vi "Close.vi"(8 "error in (no error)":errorcluster, 11 "Pump Calibration Config in":T1={"Settings"={"Cycle Period"=500.0, "Ismatech"={"VISA resource name"="", "Simulated?"=TRUE, "Pump Number"=1.0, "Reverse?"=FALSE}, "Masterflex"={"VISA resource name"="", "Simulated?"=TRUE, "Pump Number"=1.0, "Reverse?"=FALSE}, "Bronkhorst M13 Settings"={"VISA resource name"="", "Simulated?"=TRUE, "Smoothing Steps"=1}, "PID 2 Parameters"={"Input Device"=enum."Default", "Output Device"=enum."Default"}, "Tacmina Settings"={"Analog DAQ Task"="", "Digital DAQ Task"=""}, "KNF SIMDOS Settings"={"VISA resource name"="", "Simulated?"=TRUE}, "VICI M50 Settings"={"VISA resource name"="", "Pump ID"="", "Pump Head Vol"=0.0, "Reverse?"=FALSE, "Simulated?"=TRUE}, "FLOM Settings"={"VISA resource name"="", "Simulated?"=TRUE, "Pump Number"=0.0}, "Calibration Limits"={"Minimum (ml/min)"=0.0, "Maximum (ml/min)"=0.0, "Steps"=0.0}, "SSI PR Settings"={"VISA resource name"="", "Simulated?"=FALSE}, "Ismatech 4308 Settings"={"VISA resource name"="", "Pump Number"=1, "Channel Number"=0, "Simulated?"=TRUE, "Reverse?"=FALSE}, "Bronkhorst M14 Settings"={"VISA resource name"="", "Simulated?"=FALSE, "Smoothing Steps"=1}}, "Flowmeter Output"=0.0, "Density"=0.0, "FL Temp"=0.0, "Speed %"=0.0, "File Refnum"=refnum, "Pump On?"=enum."Not Initialized"} {"Settings"."Bronkhorst M14 Settings"."Smoothing Steps" min=1 step=1; "Settings"."Ismatech 4308 Settings"."Channel Number" min=0 max=3; "Settings"."Ismatech 4308 Settings"."Pump Number" min=1; "Settings"."Bronkhorst M13 Settings"."Smoothing Steps" min=1 step=1; "Settings"."Masterflex"."Pump Number" min=1.0 max=20.0 step=1.0; "Settings"."Ismatech"."Pump Number" min=1.0 max=20.0 step=1.0}) -> (0 "error out":errorcluster, 3 "Pump Calibration Config out":T1={"Settings"={"Cycle Period"=500.0, "Ismatech"={"VISA resource name"="", "Simulated?"=TRUE, "Pump Number"=1.0, "Reverse?"=FALSE}, "Masterflex"={"VISA resource name"="", "Simulated?"=TRUE, "Pump Number"=1.0, "Reverse?"=FALSE}, "Bronkhorst M13 Settings"={"VISA resource name"="", "Simulated?"=TRUE, "Smoothing Steps"=1}, "PID 2 Parameters"={"Input Device"=enum."Default", "Output Device"=enum."Default"}, "Tacmina Settings"={"Analog DAQ Task"="", "Digital DAQ Task"=""}, "KNF SIMDOS Settings"={"VISA resource name"="", "Simulated?"=TRUE}, "VICI M50 Settings"={"VISA resource name"="", "Pump ID"="", "Pump Head Vol"=0.0, "Reverse?"=FALSE, "Simulated?"=TRUE}, "FLOM Settings"={"VISA resource name"="", "Simulated?"=TRUE, "Pump Number"=0.0}, "Calibration Limits"={"Minimum (ml/min)"=0.0, "Maximum (ml/min)"=0.0, "Steps"=0.0}, "SSI PR Settings"={"VISA resource name"="", "Simulated?"=FALSE}, "Ismatech 4308 Settings"={"VISA resource name"="", "Pump Number"=1, "Channel Number"=0, "Simulated?"=TRUE, "Reverse?"=FALSE}, "Bronkhorst M14 Settings"={"VISA resource name"="", "Simulated?"=FALSE, "Smoothing Steps"=1}}, "Flowmeter Output"=0.0, "Density"=0.0, "FL Temp"=0.0, "Speed %"=0.0, "File Refnum"=refnum, "Pump On?"=enum."Not Initialized"} {"Settings"."Bronkhorst M14 Settings"."Smoothing Steps" min=1 step=1; "Settings"."Ismatech 4308 Settings"."Channel Number" min=0 max=3; "Settings"."Ismatech 4308 Settings"."Pump Number" min=1; "Settings"."Bronkhorst M13 Settings"."Smoothing Steps" min=1 step=1; "Settings"."Masterflex"."Pump Number" min=1.0 max=20.0 step=1.0; "Settings"."Ismatech"."Pump Number" min=1.0 max=20.0 step=1.0})   [LabVIEW 2018, in "Calibration.lvlib" / "Engine.lvlib"]
uses:
  Engine.lvlib
  Pump Calibration Config.ctl
  Pfizer Timed Seq/Software/Ismatec ISM 831C/Controls/Ismatech ISM831C Settings Cluster.ctl
  Pfizer Timed Seq/Software/Masterflex 7550-30/Controls/Settings Cluster.ctl
  Pfizer Timed Seq/Software/Bronkhorst M13 Flow Meter/Settings Cluster.ctl
  Pfizer Timed Seq/Software/Measure Instrument/PID Input Enum.ctl
  Pfizer Timed Seq/Software/Measure Instrument/PID 2 Output Enum.ctl
  Pfizer Timed Seq/Software/Tacmina QI/Tacmina QI DAQ Setting.ctl
  Pfizer Timed Seq/Software/KNF Pump/Settings Cluster plus SIMDOS.ctl
  Pfizer Timed Seq/Software/VICI M50 Party Mode/Settings Cluster.ctl
  Pfizer Timed Seq/Software/FLOM Pump/Settings Cluster.ctl
  Pfizer Timed Seq/Software/SSI PR Class/SSI PR or LD Settings Cluster.ctl
  Pfizer Timed Seq/Software/Ismatec 78001/Ismatec 4083.ctl
  Pfizer Timed Seq/Software/Bronkhorst M14 Flow Meter/Settings Cluster.ctl
  Pfizer Timed Seq/Software/Bronkhorst M13 Flow Meter/Bronkhorst M13 Flow Meter.lvlib
  Pfizer Timed Seq/Software/Bronkhorst M14 Flow Meter/Bronkhorst M14 Flow Meter.lvlib
  Pfizer Timed Seq/Software/Ismatec ISM 831C/Ismatec ISM 831C.lvlib
  Pfizer Timed Seq/Software/Masterflex 7550-30/Masterflex 7550-30.lvlib
  Pfizer Timed Seq/Software/VICI M50 Party Mode/VICI M6 M50 Party Mode.lvlib
  Pfizer Timed Seq/Software/Tacmina QI/Tacmina QI.lvlib
  Pfizer Timed Seq/Software/KNF Pump/KNF SIMDOS.lvlib
  Pfizer Timed Seq/Software/FLOM Pump/FLOM Pump.lvlib
  Pfizer Timed Seq/Software/SSI PR Class/SSI PR or LD Pump.lvlib
  Pfizer Timed Seq/Software/Ismatec 78001/Ismatec 4308.lvlib
  Pfizer Timed Seq/Software/Calibration VIs/Calibration.lvlib
panel:
  # "Output Instruments"
  # "Input Instruments"
  # "Output Instruments"
  # "Input Instruments"
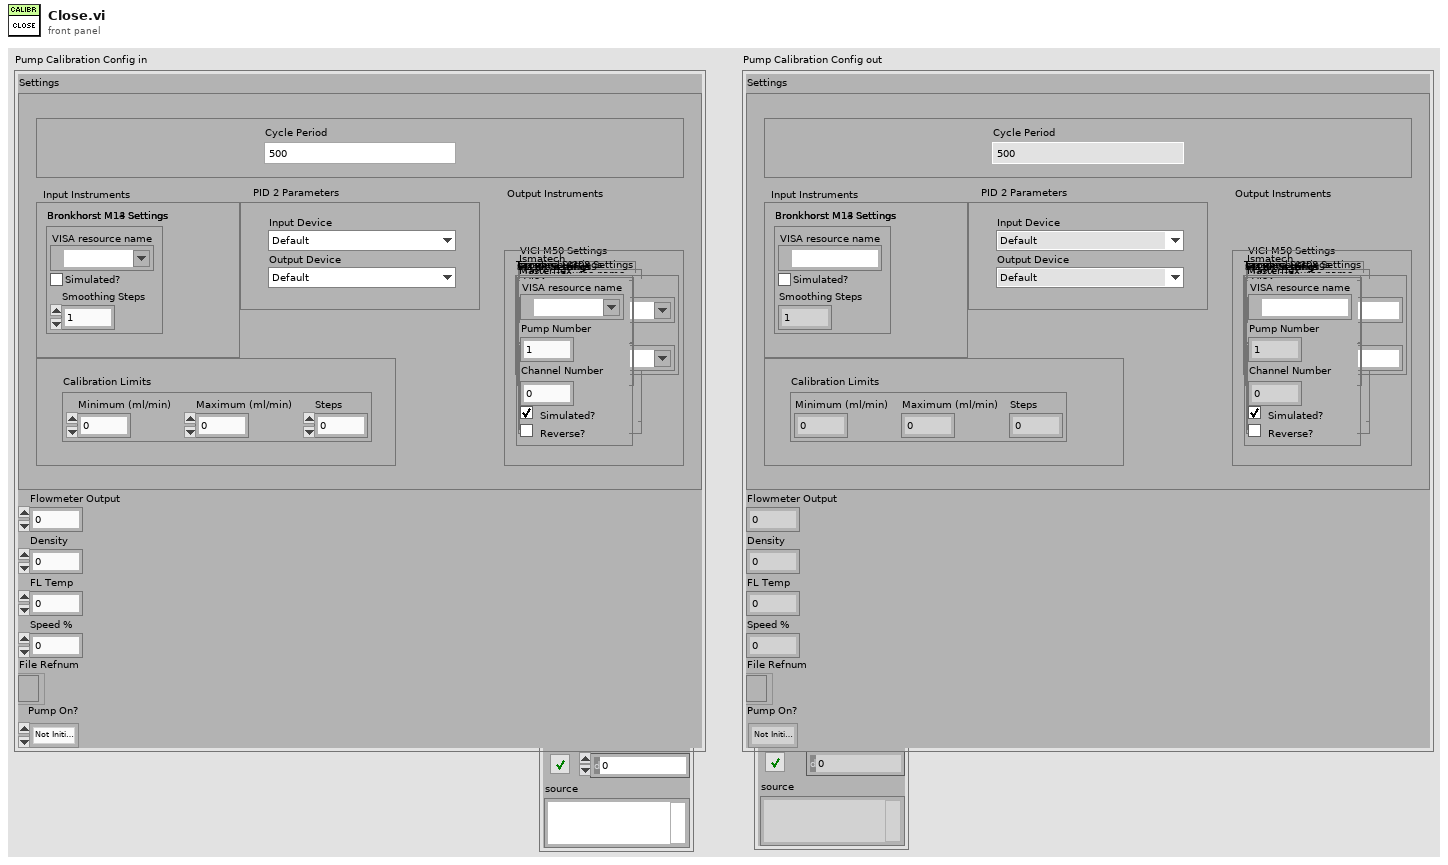
[diagram p1: front panel]
types:
  T1 = typedef "Calibration.lvlib/Pump Calibration Config.ctl" = cluster{"Settings":cluster{"Cycle Period":dbl, "Ismatech":T2, "Masterflex":T3, "Bronkhorst M13 Settings":T4, "PID 2 Parameters":cluster{"Input Device":T5, "Output Device":T6}, "Tacmina Settings":T7, "KNF SIMDOS Settings":T8, "VICI M50 Settings":T9, "FLOM Settings":T10, "Calibration Limits":cluster{"Minimum (ml/min)":dbl, "Maximum (ml/min)":dbl, "Steps":dbl}, "SSI PR Settings":T11, "Ismatech 4308 Settings":T12, "Bronkhorst M14 Settings":T13}, "Flowmeter Output":dbl, "Density":dbl, "FL Temp":dbl, "Speed %":dbl, "File Refnum":refnum<file>, "Pump On?":enum16{"Off", "On", "Not Initialized"}}
  T2 = typedef "Ismatec ISM 831C.lvlib/Ismatech ISM831C Settings Cluster.ctl" = cluster{"VISA resource name":refnum<visa-resource-name>, "Simulated?":bool, "Pump Number":dbl, "Reverse?":bool}
  T3 = typedef "Masterflex 7550-30.lvlib/Settings Cluster.ctl" = cluster{"VISA resource name":refnum<visa-resource-name>, "Simulated?":bool, "Pump Number":dbl, "Reverse?":bool}
  T4 = typedef "Bronkhorst M13 Flow Meter.lvlib/Settings Cluster.ctl" = cluster{"VISA resource name":refnum<visa-resource-name>, "Simulated?":bool, "Smoothing Steps":i32}
  T5 = typedef "PID Input Enum.ctl" = enum16{"Default", "Bronkhorst M13", "Bronkhorst M14", "Scale Rate of Change"}
  T6 = typedef "PID 2 Output Enum.ctl" = enum16{"Default", "Ismatec ISM 4308", "Ismatec ISM 831C", "Masterflex 7550-30", "VICI M6", "VICI M50", "Tacmina QI", "KNF SIMDOS", "ASIA Type C", "FLOM UI-22-11", "SSI PR/LD", "SSI P40", "Masterflex 75211-70"}
  T7 = typedef "Tacmina QI.lvlib/Tacmina QI DAQ Setting.ctl" = cluster{"Analog DAQ Task":refnum<k21>, "Digital DAQ Task":refnum<k21>}
  T8 = typedef "KNF SIMDOS.lvlib/Settings Cluster plus SIMDOS.ctl" = cluster{"VISA resource name":refnum<visa-resource-name>, "Simulated?":bool}
  T9 = typedef "VICI M6 M50 Party Mode.lvlib/Settings Cluster.ctl" = cluster{"VISA resource name":refnum<visa-resource-name>, "Pump ID":string, "Pump Head Vol":dbl, "Reverse?":bool, "Simulated?":bool}
  T10 = typedef "FLOM Pump.lvlib/Settings Cluster.ctl" = cluster{"VISA resource name":refnum<visa-resource-name>, "Simulated?":bool, "Pump Number":dbl}
  T11 = typedef "SSI PR or LD Pump.lvlib/SSI PR or LD Settings Cluster.ctl" = cluster{"VISA resource name":refnum<visa-resource-name>, "Simulated?":bool}
  T12 = typedef "Ismatec 4308.lvlib/Ismatec 4083.ctl" = cluster{"VISA resource name":refnum<visa-resource-name>, "Pump Number":i16, "Channel Number":i16, "Simulated?":bool, "Reverse?":bool}
  T13 = typedef "Bronkhorst M14 Flow Meter.lvlib/Settings Cluster.ctl" = cluster{"VISA resource name":refnum<visa-resource-name>, "Simulated?":bool, "Smoothing Steps":i32}
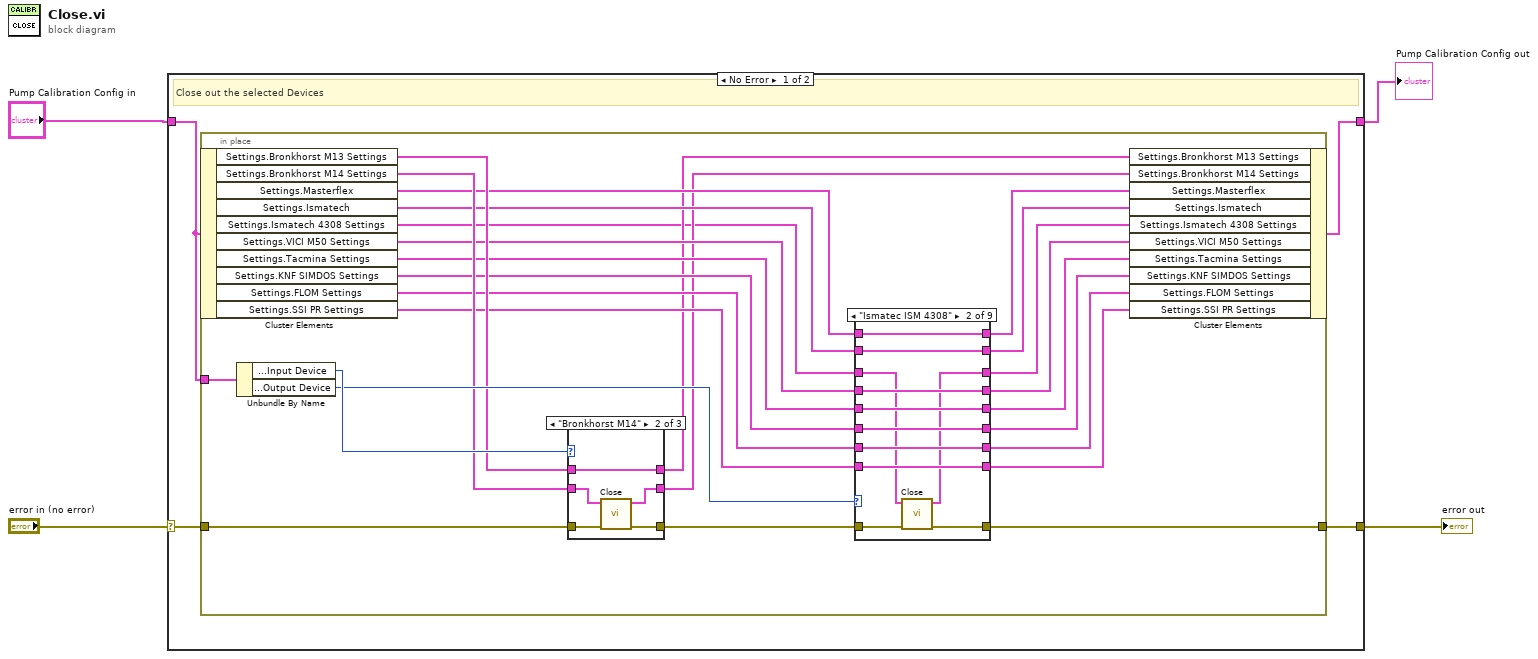
[diagram p0: block diagram]
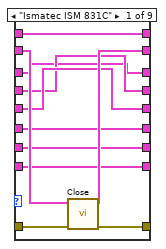
[diagram p2: hidden frame]
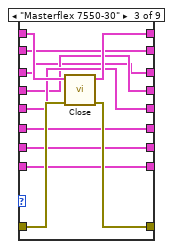
[diagram p3: hidden frame]
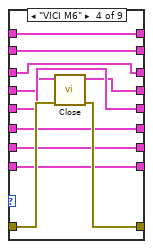
[diagram p4: hidden frame]
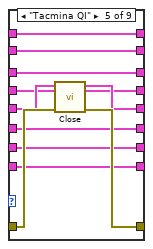
[diagram p5: hidden frame]
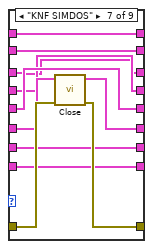
[diagram p7: hidden frame]
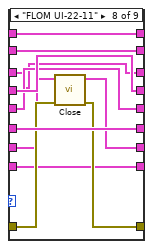
[diagram p8: hidden frame]
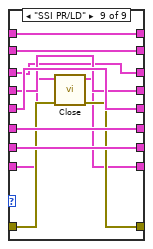
[diagram p9: hidden frame]
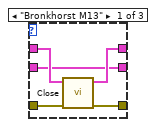
[diagram p10: hidden frame]
diagram:
  n1 = case shown="No Error" "error in (no error)" {
    selector: "error in (no error)" -> [w8 w146]
    tunnel: [w7 w146] -> w3
    tunnel: "Pump Calibration Config in" -> [w6 w145]
    tunnel: [w5 w145] -> w2
    frame No Error {
      # "Close out the selected Devices"
      n2 = in-place {
        in-place-border: w8 -> [w33]
        in-place-border: [w32] -> w7
        in-place-border: w6 -> [w29]
        n3 = in-place-cluster #1(w6) -> ("Settings.Bronkhorst M13 Settings"=w28:T4, "Settings.Bronkhorst M14 Settings"=w27:T13, "Settings.Masterflex"=w26:T3, "Settings.Ismatech"=w25:T2, "Settings.Ismatech 4308 Settings"=w10:T12, "Settings.VICI M50 Settings"=w24:T9, "Settings.Tacmina Settings"=w23:T7, "Settings.KNF SIMDOS Settings"=w22:T8, "Settings.FLOM Settings"=w21:T10, "Settings.SSI PR Settings"=w20:T11)
        n4 = Unbundle By Name(w29) -> ("Settings.PID 2 Parameters.Input Device"=w34:T5, "Settings.PID 2 Parameters.Output Device"=w30:T6)
        n5 = case shown="\"Bronkhorst M14\"" w34 {
          tunnel: w28 -> [w134 w139 w144]
          tunnel: w33 -> [w136 w141 w143]
          tunnel: [w135 w140 w143] -> w31
          tunnel: [w133 w139 w144] -> w19
          tunnel: w27 -> [w132 w138 w142]
          tunnel: [w132 w137 w142] -> w18
          frame "Bronkhorst M13" {
            n6 = call "Close.vi"("error in (no error)"=w136, "Bronkhorst Settings in"=w134) -> ("error out"=w135:errorcluster, "Bronkhorst Settings out"=w133:T4)  [unwired: 8 in]
          }
          frame "Bronkhorst M14" {
            n7 = call "Close.vi"("error in (no error)"=w141, "Bronkhorst Settings in"=w138) -> ("error out"=w140:errorcluster, "Bronkhorst Settings out"=w137:T13)  [unwired: 8 in]
          }
          frame "Default", Default {
          }
        }
        n8 = case shown="\"Ismatec ISM 4308\"" w30 {
          tunnel: w26 -> [w41 w56 w67 w75 w86 w98 w109 w120 w131]
          tunnel: [w41 w56 w66 w75 w86 w98 w109 w120 w131] -> w17
          tunnel: w25 -> [w43 w55 w64 w76 w87 w97 w108 w119 w130]
          tunnel: [w45 w48 w65 w77 w88 w96 w105 w114 w124] -> w32
          tunnel: w31 -> [w44 w49 w63 w78 w89 w96 w106 w115 w125]
          tunnel: [w42 w55 w64 w76 w87 w97 w108 w119 w130] -> w16
          tunnel: [w40 w54 w62 w74 w85 w95 w107 w117 w129] -> w14
          tunnel: w23 -> [w40 w54 w62 w74 w84 w95 w107 w117 w129]
          tunnel: [w39 w53 w61 w73 w83 w94 w104 w116 w128] -> w13
          tunnel: w22 -> [w39 w53 w61 w73 w83 w94 w103 w116 w128]
          tunnel: [w38 w52 w60 w72 w82 w93 w102 w118 w127] -> w15
          tunnel: w24 -> [w38 w52 w60 w71 w82 w93 w102 w118 w127]
          tunnel: [w37 w51 w59 w70 w81 w92 w101 w112 w126] -> w12
          tunnel: w21 -> [w37 w51 w59 w70 w81 w92 w101 w113 w126]
          tunnel: w20 -> [w36 w50 w58 w69 w80 w91 w100 w111 w123]
          tunnel: [w36 w50 w58 w69 w80 w91 w100 w111 w122] -> w11
          tunnel: w10 -> [w35 w47 w57 w68 w79 w90 w99 w110 w121]
          tunnel: [w35 w46 w57 w68 w79 w90 w99 w110 w121] -> w9
          frame "Ismatec ISM 831C" {
            n9 = call "Close.vi"("error in (no error)"=w44, "Ismatech Settings"=w43) -> ("error out"=w45:errorcluster, "Ismatech Settings"=w42:T2)  [unwired: 7 in, 1 out]
          }
          frame "Ismatec ISM 4308" {
            n10 = call "Close.vi"("error in (no error)"=w49, "Ismatech 3 Channel Settings In"=w47) -> ("error out"=w48:errorcluster, "Ismatech 3 Channel Settings Out"=w46:T12)  [unwired: 7 in, 1 out]
          }
          frame "Masterflex 7550-30" {
            n11 = call "Close.vi"("error in (no error)"=w63, "Masterflex Settings in"=w67) -> ("error out"=w65:errorcluster, "Masterflex Settings out"=w66:T3)  [unwired: 7 in, 1 out]
          }
          frame "VICI M6" {
            n12 = call "Close.vi"("error in (no error)"=w78, "VICI Settings"=w71) -> ("error out"=w77:errorcluster, "VICI Settings"=w72:T9)  [unwired: 7 in, 1 out]
          }
          frame "Tacmina QI" {
            n13 = call "Close.vi"("error in"=w89, "Tacmina Settings in"=w84) -> ("error out"=w88:errorcluster, "Tacmina Settings out"=w85:T7)  [unwired: 8 in]
          }
          frame "Default", Default {
          }
          frame "KNF SIMDOS" {
            n14 = call "Close.vi"("error in (no error)"=w106, "KNF Settings"=w103) -> ("error out"=w105:errorcluster, "KNF Settings"=w104:T8)  [unwired: 7 in, 1 out]
          }
          frame "FLOM UI-22-11" {
            n15 = call "Close.vi"("error in (no error)"=w115, "FLOM Settings in"=w113) -> ("error out"=w114:errorcluster, "FLOM Settings out"=w112:T10)  [unwired: 7 in, 1 out]
          }
          frame "SSI PR/LD" {
            n16 = call "Close.vi"("error in (no error)"=w125, "SSI PR Settings In"=w123) -> ("error out"=w124:errorcluster, "SSI PR Settings Out"=w122:T11)  [unwired: 7 in, 1 out]
          }
        }
        n17 = in-place-cluster #1("Settings.Bronkhorst M13 Settings"=w19, "Settings.Bronkhorst M14 Settings"=w18, "Settings.Masterflex"=w17, "Settings.Ismatech"=w16, "Settings.Ismatech 4308 Settings"=w9, "Settings.VICI M50 Settings"=w15, "Settings.Tacmina Settings"=w14, "Settings.KNF SIMDOS Settings"=w13, "Settings.FLOM Settings"=w12, "Settings.SSI PR Settings"=w11) -> (w5:T1)
      }
    }
    frame Error {
    }
  }
  "error out" <- w3
  "Pump Calibration Config out" <- w2
